vi "hydrolysis_reactor_run.vi"(10 "spec_file":path) -> (2 "hydrolysis_path":path)   [LabVIEW 2019]
uses:
  <vilib>/Utility/sysdir.llb/System Directory Type.ctl
  lib/libSimulationControl/libSimulationControl.lvlib
panel:
  # "*******************************************************************\nBiogas Plant Control\n\nAuthor: Paul Zügel\nGCSC-Frankfurt am Main 2020\n\n*******************************************************************"
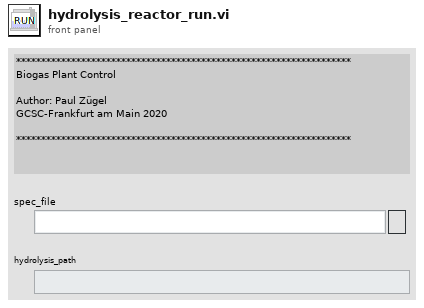
[diagram p1: front panel]
types:
  T1 = typedef "System Directory Type.ctl" = i32
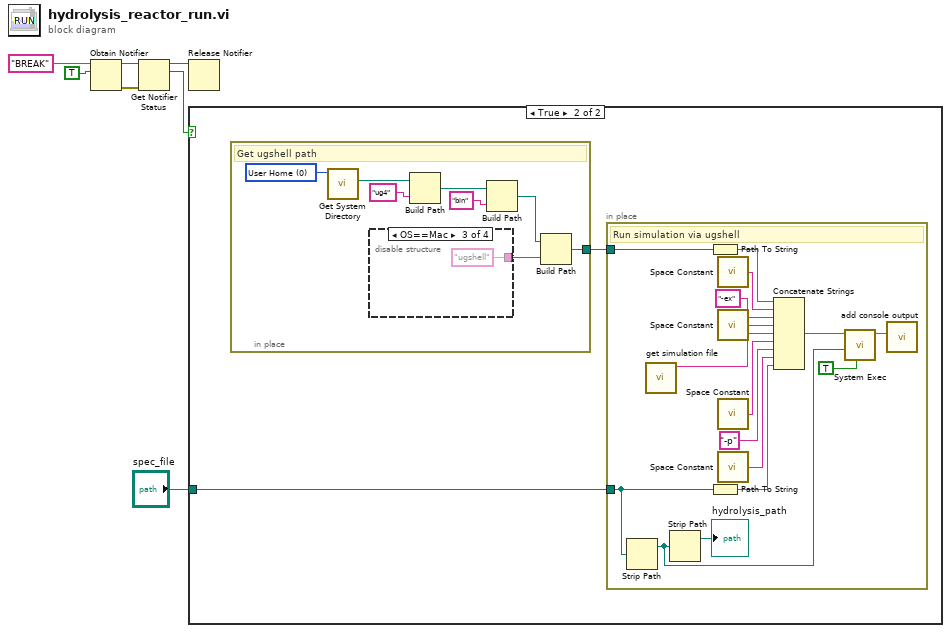
[diagram p0: block diagram]
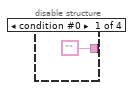
[diagram p3: hidden frame]
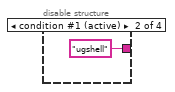
[diagram p4: hidden frame]
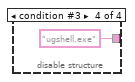
[diagram p5: hidden frame]
diagram:
  n1 = Obtain Notifier(name (unnamed)="BREAK", notification data type=TRUE) -> (notifier out=w5:refnum<notifier>, error out=w4:errorcluster)  [unwired: 2 in, 1 out]
  n2 = Get Notifier Status(notifier=w5, error in (no error)=w4) -> (notifier out=w1:refnum<notifier>, current notification=w3:bool)  [unwired: 3 out]
  n3 = Release Notifier(notifier=w1) -> ()  [unwired: 2 in, 3 out]
  n4 = case shown="True" w3 {
    tunnel: "spec_file" -> [_ w9]
    frame False {
    }
    frame True {
      # "Define current paths"
      # "True only on first Iteration (current_time = starttime)\nWe get all names of output Files from the outputFiles.lua and copy them from tmp to the working directory."
      n5 = in-place {
        in-place-border: [w10] -> w8
        w11 = T1 0 items=["User Home"=0, "User Desktop"=1, "User Documents"=2, "User Application Data"=3, "User Preferences"=4, "User Temporary"=5, "Public Documents"=6, "Public Application Data"=7, "Public Preferences"=8, "Public Cache"=13, "System Core Libraries"=9, "System Installed Libraries"=10, "Application Files"=11, "Boot Volume Root"=12] ("system directory type")
        # "Get ugshell path"
        n6 = call <vilib>:"Get System Directory.vi"("system directory type"=w11) -> ("system directory"=w14:path)  [unwired: 10 in]
        n7 = disable-structure shown="OS==Mac" {
          disable-tunnel: ["" "ugshell" ("name or relative path") "ugshell" ("name or relative path") "ugshell.exe" ("name or relative path")] -> w17
          frame condition #0 {
          }
          frame condition #1 (active) {
          }
          frame condition #2 {
          }
          frame condition #3 {
          }
        }
        n8 = Build Path(base path=w14, name or relative path="ug4") -> (appended path=w15:path)
        n9 = Build Path(base path=w15, name or relative path="bin") -> (appended path=w16:path)
        n10 = Build Path(base path=w16, name or relative path=w17) -> (appended path=w10:path)
      }
      n11 = in-place {
        in-place-border: w9 -> [w27]
        in-place-border: w8 -> [w23]
        # "Run simulation via ugshell"
        n12 = Strip Path(path=w27) -> (stripped path=w25:path)  [unwired: 1 out]
        n13 = call "get simulation file.vi"() -> ("function return"=w29:string)  [unwired: 10 in, 1 out]
        n14 = Strip Path(path=w25) -> (stripped path=→"hydrolysis_path":path)  [unwired: 1 out]
        n15 = Path To String(path=w23) -> (string=w22:string)
        n16 = Path To String(path=w27) -> (string=w26:string)
        n17 = call <vilib>:"Space Constant.vi"() -> ("String"=w32:string)
        n18 = call <vilib>:"Space Constant.vi"() -> ("String"=w33:string)
        n19 = call <vilib>:"Space Constant.vi"() -> ("String"=w34:string)
        n20 = call <vilib>:"Space Constant.vi"() -> ("String"=w36:string)
        n21 = Concatenate Strings(w22, w32, "-ex" ("command line"), w33, w29, w34, "-p" ("command line"), w36, w26) -> (w35:string)
        n22 = call <vilib>:"System Exec.vi"("run minimized? (F)"=TRUE, "working directory"=w25, "command line"=w35) -> ("standard output"=w37:string)  [unwired: 5 in, 3 out]
        n23 = call "add console output.vi"("add_to_console"=w37) -> ()  [unwired: 11 in]
      }
    }
  }
